vi "Queue Self SubVI.vi"(4 "Priority?":bool, 6 "Msg Strategy":refnum<class "Msg Strategy.lvclass">, 9 "Queue Mailbox":refnum<data-value>, 10 "jettl in":refnum<class "jettl.lvclass">) -> (2 "jettl out":refnum<class "jettl.lvclass">)   [LabVIEW 2021, in "jettl.lvlib"]
uses:
  jettl.lvlib
  jettl/jettl.lvclass
  Msg Strategy/Msg Strategy.lvclass
  Queue Mailbox/Queue Mailbox.lvclass
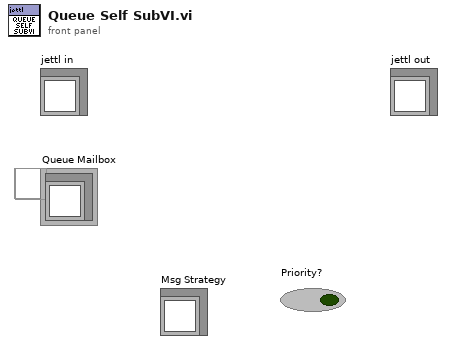
[diagram p1: front panel]
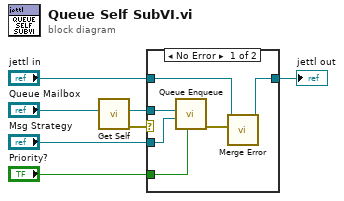
[diagram p0: block diagram]
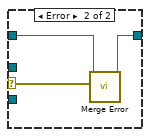
[diagram p2: hidden frame]
diagram:
  n1 = call "Get Self.vi"("Queue Mailbox"="Queue Mailbox") -> ("error out"=w4:errorcluster, "Self"=w5:refnum<data-value>)  [unwired: 9 in]
  n2 = case shown="No Error" w4 {
    selector: w4 -> [_ w15]
    tunnel: "Priority?" -> [w12 _]
    tunnel: "Msg Strategy" -> [w11 _]
    tunnel: "jettl in" -> [w10 w14]
    tunnel: [w9 w16] -> w2
    tunnel: w5 -> [w8 _]
    frame No Error {
      n3 = call "Queue Enqueue.vi"("Priority?"=w12, "Msg Strategy"=w11, "Queue"=w8) -> ("error out"=w13:errorcluster)  [unwired: 8 in]
      n4 = call-dynamic "Merge Error.vi"("Error"=w13, "Merge Error in"=w10) -> ("Merge Error out"=w9:refnum<class "jettl.lvclass">)  [unwired: 9 in]
    }
    frame Error {
      n5 = call-dynamic "Merge Error.vi"("Error"=w15, "Merge Error in"=w14) -> ("Merge Error out"=w16:refnum<class "jettl.lvclass">)  [unwired: 9 in]
    }
  }
  "jettl out" <- w2
